vi "Open File.vi"(0 "reference in":refnum<class "RPC.lvclass">, 5 "error in (no error)":errorcluster, 6 "IO Type":enum16{"READ File", "WRITE File"}(ring), 7 "MegaDAC RPC File (*.rsp)":path) -> (13 "file or folder exists?":bool, 14 "reference out":refnum<class "RPC.lvclass">, 19 "error out":errorcluster)   [LabVIEW 2020, in "RPC.lvclass"]
uses:
  RPC.lvclass
  API/Generic Utilities_class/Generic Utilities.lvclass
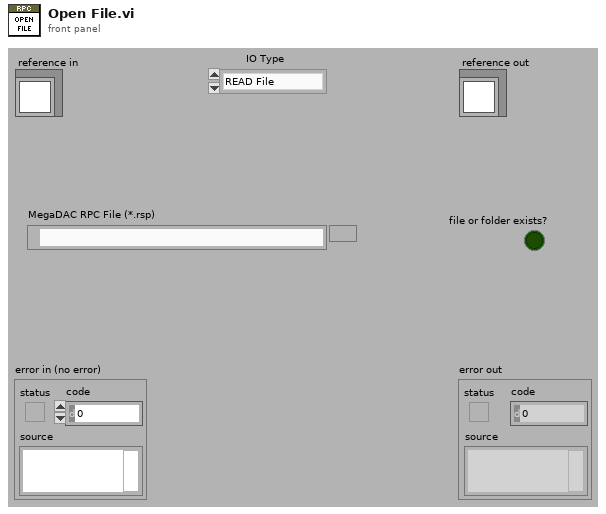
[diagram p1: front panel]
types:
  T1 = enum16{"open", "replace", "create", "open or create", "replace or create", "replace or create with confirmation"}
  T2 = typedef "RPC.lvclass/ObjectAttributesRef.ctl" = refnum<data-value>
  T3 = typedef "RPC.lvclass/ObjectAttributes.ctl" = cluster{"File Refnum":refnum<file>, "File total size":i32, "Offset from start of file":i32, "Time Type":enum16{"Response", "Drive"}, "Full Scale":dbl[unit], "New Time Data Obj?":bool, "Header":cluster{"Num Header":i32, "Num Parameter":i32, "Nb Channels":i32, "dT":dbl, "Number of Groups":i32, "Group size":i32, "Units":string[], "Names":string[], "Sensitivity":dbl[], "Complete header":string[]}, "Time Data":refnum<class "GSwFormDSP.lvclass">}
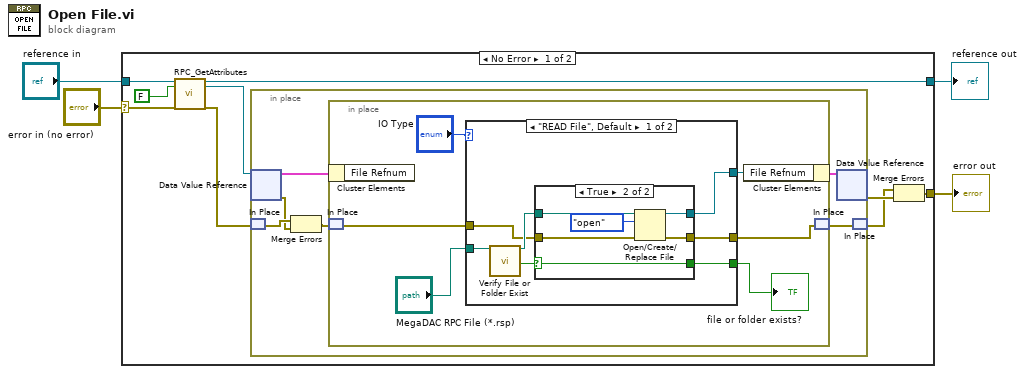
[diagram p0: block diagram]
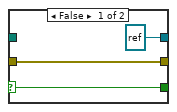
[diagram p2: hidden frame]
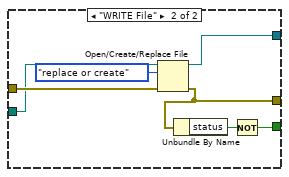
[diagram p3: hidden frame]
diagram:
  n1 = case shown="No Error" "error in (no error)" {
    selector: "error in (no error)" -> [w9 w50]
    tunnel: [w13 w50] -> w3
    tunnel: [w8 w49] -> w1
    tunnel: "reference in" -> [w11 w49]
    frame No Error {
      n2 = call "RPC_GetAttributes.vi"("reference in"=w11, "return data? (T)"=FALSE, "error in (no error)"=w9) -> ("reference out"=w8:refnum<class "RPC.lvclass">, "attributes ref"=w7:T2, "error out"=w6:errorcluster)  [unwired: 13 in, 1 out]
      n3 = in-place {
        n4 = in-place-dvr #1(w7) -> (w18:T3, w16:errorcluster)
        n5 = in-place-match #2(w6) -> (w17:errorcluster)
        n6 = Merge Errors(w17, w16) -> (w14:errorcluster)
        n7 = in-place {
          n8 = in-place-cluster #3(w18) -> ()  [unwired: 1 out]
          n9 = in-place-match #4(w14) -> (w22:errorcluster)
          n10 = case shown="\"READ File\", Default" "IO Type" {
            tunnel: "MegaDAC RPC File (*.rsp)" -> [w32 w47]
            tunnel: [w30 w45] -> w24
            tunnel: [w29 w44] -> w23
            tunnel: w22 -> [w28 w48]
            tunnel: [w26 w43] -> w21
            frame "READ File", Default {
              n11 = call "Verify File or Folder Exist.vi"("path"=w32) -> ("dup path"=w31:path, "file or folder exists?"=w27:bool)  [unwired: 16 in, 1 out]
              n12 = case shown="True" w27 {
                selector: w27 -> [w33 w36]
                tunnel: w31 -> [_ w41]
                tunnel: [refnum<file> refnum ("refnum out") w40] -> w30
                tunnel: [w34 w38] -> w29
                tunnel: w28 -> [w34 w37]
                tunnel: [w33 w36] -> w26
                frame False {
                }
                frame True {
                  n13 = Open/Create/Replace File(file path (use dialog)=w41, error in=w37, operation (0:open)=T1."open") -> (refnum out=w40:refnum<file>, error out=w38:errorcluster)  [unwired: 3 in, 1 out]
                }
              }
            }
            frame "WRITE File" {
              n14 = Open/Create/Replace File(file path (use dialog)=w47, error in=w48, operation (0:open)=T1."replace or create") -> (refnum out=w45:refnum<file>, error out=w44:errorcluster)  [unwired: 3 in, 1 out]
              n15 = Unbundle By Name(w44) -> ("status"=w42:bool)
              n16 = Not(x=w42) -> (.not. x?=w43:bool)
            }
          }
          "file or folder exists?" <- w21
          n17 = in-place-cluster #3("File Refnum"=w24) -> (w19:T3)
          n18 = in-place-match #4(w23) -> (w15:errorcluster)
        }
        n19 = in-place-dvr #1(w19) -> (w12:errorcluster)  [unwired: 1 out]
        n20 = in-place-match #2(w15) -> (w5:errorcluster)
      }
      n21 = Merge Errors(w5, w12) -> (w13:errorcluster)
    }
    frame Error {
    }
  }
  "error out" <- w3
  "reference out" <- w1
